vi "Shared Variable Container Filename--Const.vi"() -> (3 "Shared Variables Container Filename":string="DTACQ - Network Enabled Device Driver.lvlib")   [LabVIEW 2017, in "Shared Variables Library.lvlib"]
doc: "The filename of the shared variable container."
uses:
  Shared Variables Library.lvlib
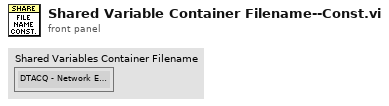
[diagram p1: front panel]
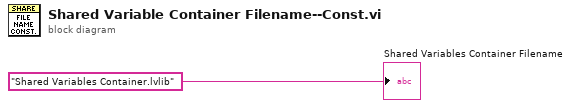
[diagram p0: block diagram]
diagram:
  "Shared Variables Container Filename" <- "Shared Variables Container.lvlib"
